vi "ConfigMessageMetadata.vi"(7 "{{Name}}Message":refnum<class "{{Name}}Message.lvclass">, 9 "ActorLifetime":T2, 10 "ActorRelation":T1, 11 "ActorAlias":string) -> (5 "{{Name}}Message":refnum<class "{{Name}}Message.lvclass">)   [LabVIEW 2020, in "_Template.lvlib" / "Templates.lvlib" / "{{Name}}Message.lvlib" / "{{Name}}Message.lvclass"]
uses:
  {{Name}}Message.lvclass
  {{Name}}Message.lvclass/{{Name}}Message.ctl
  jettl/jettl/jettl.lvlib
  jettl/jettl/ActorLifetime.ctl
  jettl/jettl/ActorRelation.ctl
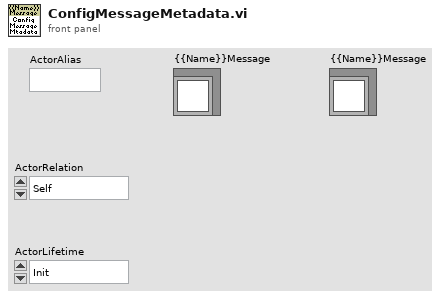
[diagram p1: front panel]
types:
  T1 = typedef "jettl.lvlib/ActorRelation.ctl" = enum16{"Self", "Actor"}
  T2 = typedef "jettl.lvlib/ActorLifetime.ctl" = enum16{"Init", "Spawn", "Setup", "Teardown Before Running", "Running", "Stop Called", "Stopping With Children", "Stopping Without Children", "Teardown After Running", "Stopped"}
  T3 = typedef "jettl.lvlib/MessageMetadata.ctl" = cluster{"ActorAlias":string, "ActorRelation":T1, "ActorLifetime":T2, "AbsoluteTime":timestamp, "RelativeTime":dbl}
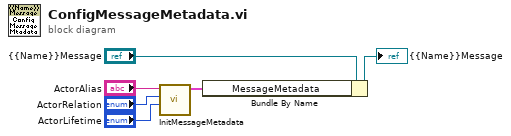
[diagram p0: block diagram]
diagram:
  n1 = call "InitMessageMetadata.vi"("ActorLifetime"="ActorLifetime", "ActorRelation"="ActorRelation", "ActorAlias"="ActorAlias") -> ("MessageMetadata"=w4:T3)  [unwired: 8 in]
  n2 = Bundle By Name(cluster="{{Name}}Message", "MessageMetadata"=w4) -> (→"{{Name}}Message":refnum<class "{{Name}}Message.lvclass">)
